vi "Power_Supply Close References.vi"(8 "error in (no error)":errorcluster, 11 "User Reference":T1) -> (0 "error out":errorcluster)   [LabVIEW 2018, in "Power_Supply Virtual.lvclass"]
uses:
  Power_Supply Virtual.lvclass
  Controls/User Reference.ctl
  Power_Supply Global.vi
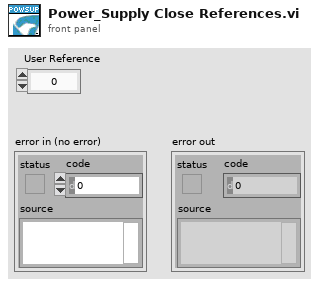
[diagram p1: front panel]
types:
  T1 = typedef "User Reference.ctl" = i32
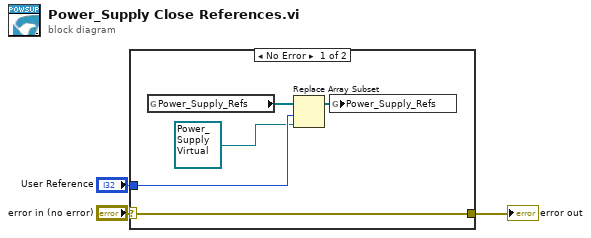
[diagram p0: block diagram]
diagram:
  n1 = case shown="No Error" "error in (no error)" {
    selector: "error in (no error)" -> [w8 w9]
    tunnel: [w8 w9] -> w2
    tunnel: "User Reference" -> [w6 _]
    frame No Error {
      n2 = global read "Power_Supply Global.vi" "Power_Supply_Refs"() -> (w7:refnum<class "Power_Supply Virtual.lvclass">[])
      n3 = Replace Array Subset(array=w7, new element=refnum<class "Power_Supply Virtual.lvclass"> refnum ("Power_Supply Virtual.lvclass"), index=w6) -> (w5:refnum<class "Power_Supply Virtual.lvclass">[])
      n4 = global write "Power_Supply Global.vi" "Power_Supply_Refs"(w5) -> ()
    }
    frame Error {
    }
  }
  "error out" <- w2
